vi "Run VIA.vi"(6 "Buildlog":path, 8 "error in (no error)":errorcluster, 10 "args":string[](array[string]), 11 "VI Path":path) -> (0 "error out":errorcluster)   [LabVIEW 2010]
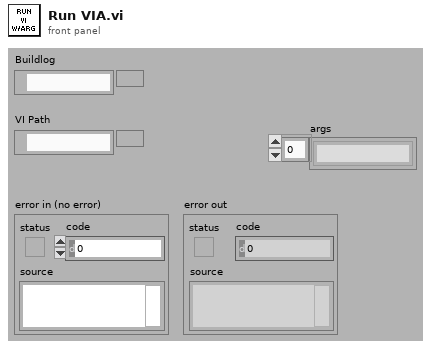
[diagram p1: front panel]
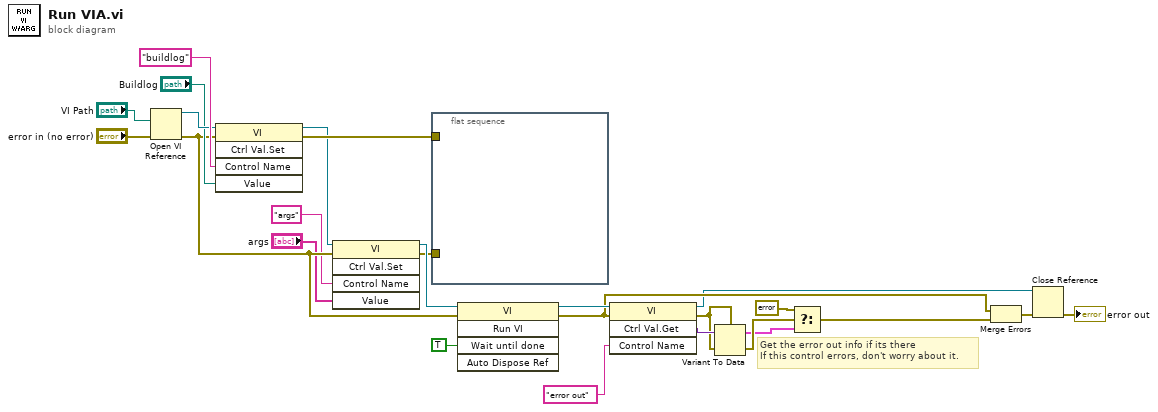
[diagram p0: block diagram]
diagram:
  # "Get the error out info if its there\nIf this control errors, don't worry about it."
  n1 = Open VI Reference(vi path="VI Path", error in (no error)="error in (no error)") -> (vi reference=w9:refnum<vi>, error out=w4:errorcluster)  [unwired: 4 in]
  n2 = invoke class="VI" method="Ctrl Val.Set"(reference=w9, error in=w4, "Control Name"="buildlog", "Value"="Buildlog") -> (reference out=w5:refnum<vi>, error out=w7:errorcluster)  [unwired: 1 in, 3 out]
  n3 = invoke class="VI" method="Ctrl Val.Set"(reference=w5, error in=w4, "Control Name"="args", "Value"="args") -> (reference out=w6:refnum<vi>, error out=w3:errorcluster)  [unwired: 1 in, 3 out]
  n4 = flat-sequence {
    tunnel: w7 -> [_]
    tunnel: w3 -> [_]
    frame #0 {
    }
  }
  n5 = invoke class="VI" method="Run VI"(reference=w6, error in=w4, "Wait until done"=TRUE ("Wait Until Done")) -> (reference out=w22:refnum<vi>, error out=w15:errorcluster)  [unwired: 2 in, 3 out]
  n6 = invoke class="VI" method="Ctrl Val.Get"(reference=w22, error in=w15, "Control Name"="error out") -> (reference out=w11:refnum<vi>, error out=w19:errorcluster, "Get Control Value Variant"=w20:variant)  [unwired: 1 in, 1 out]
  n7 = Variant To Data(error in=w19, Variant=w20, type=w19) -> (error out=w18:errorcluster, data=w16:cluster{})
  n8 = Select(t=errorcluster {"status"=FALSE, "code"=0, "source"=""}, s=w18, f=w16) -> (s? t:f=w14:errorcluster)
  n9 = Merge Errors(w15, w14) -> (w13:errorcluster)
  n10 = Close Reference(reference=w11, error in (no error)=w13) -> (error out=→"error out":errorcluster)
